vi "DriveShifter.vi"(8 "error in (no error)":errorcluster, 10 "HighGear?":bool, 11 "Pod Drive in":refnum<class "Pod Drive.lvclass">) -> (0 "error out":errorcluster, 3 "Pod Drive out":refnum<class "Pod Drive.lvclass">)   [LabVIEW 2018, in "Drive.lvlib" / "Pod Drive.lvclass"]
doc: "Shifts drive into high gear and adjusts PIDF slots"
uses:
  Pod Drive.lvclass
  Pod Drive.lvclass/Pod Drive.ctl
  Drive.lvclass
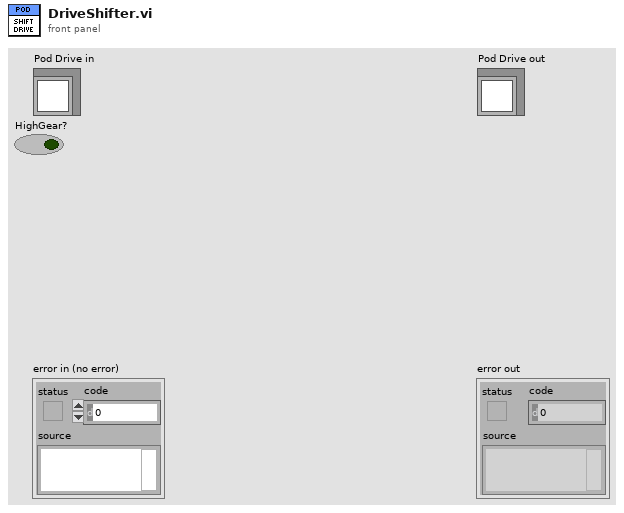
[diagram p1: front panel]
types:
  T1 = typedef "Drive.lvlib/Pod Drive.lvclass/Mode.ctl" = enum16{"ClosedLoop", "MotionMagic"}
  T2 = typedef "WPI_MotorControlDeviceRef.ctl" = cluster{"DeviceStatus":errorcluster, "Type":T3, "PWM":cluster{"PWM Channel":T4, "DeadBand":T5}, "CAN":cluster{"Device Number":u8, "SetOutput VI Ref":variant, "GetOutput VI Ref":variant, "Enable VI Ref":variant, "Disable VI Ref":variant, "Data":variant}, "Invert":bool, "DIO PWM":cluster{"PWM \"Enable\" Channel":T4, "DIOChannel":T6, "PWM Rate":dbl}}
  T3 = typedef "WPI_MotorControlType.ctl" = enum16{"PWM", "CAN", "DIO PWM"}
  T4 = typedef "FPGA_DIOPWMChannel.ctl" = enum8{"PWM 0", "PWM 1", "PWM 2", "PWM 3", "PWM 4", "PWM 5", "PWM 6", "PWM 7", "PWM 8", "PWM 9", "PWM MXP 0", "PWM MXP 1", "PWM MXP 2", "PWM MXP 3", "PWM MXP 4", "PWM MXP 5", "PWM MXP 6", "PWM MXP 7", "PWM MXP 8", "PWM MXP 9", "Invalid"}
  T5 = typedef "WPI_PWMDeadband.ctl" = cluster{"Name":string, "maxPositivePwm":i32, "minPositivePwm":i32, "centerPwm":i32, "maxNegativePwm":i32, "minNegativePwm":i32, "angularRange":u16}
  T6 = typedef "FPGA_DIOChannel.ctl" = enum8{"DIO 0", "DIO 1", "DIO 2", "DIO 3", "DIO 4", "DIO 5", "DIO 6", "DIO 7", "DIO 8", "DIO 9", "DIO MXP 0", "DIO MXP 1", "DIO MXP 2", "DIO MXP 3", "DIO MXP 4", "DIO MXP 5", "DIO MXP 6", "DIO MXP 7", "DIO MXP 8", "DIO MXP 9", "DIO MXP 10", "DIO MXP 11", "DIO MXP 12", "DIO MXP 13", "DIO MXP 14", "DIO MXP 15", "SPI Port CS1", "SPI Port CS2", "SPI Port CS3", "SPI Port MISO", "SPI Port MOSI", "Invalid"}
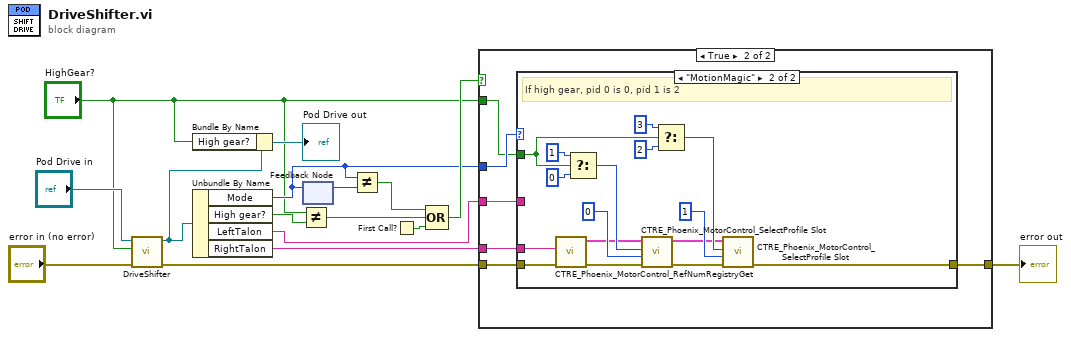
[diagram p0: block diagram]
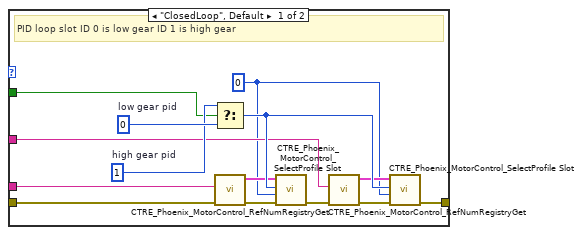
[diagram p3: hidden frame]
diagram:
  n1 = call-parent "DriveShifter.vi"("error in (no error)"="error in (no error)", "HighGear?"="HighGear?", "Drive in"="Pod Drive in") -> ("error out"=w5:errorcluster, "Drive out"=w14:refnum<class "Pod Drive.lvclass">)  [unwired: 7 in]
  n2 = Bundle By Name(cluster=w14, "High gear?"="HighGear?") -> (→"Pod Drive out":refnum<class "Pod Drive.lvclass">)
  n3 = Unbundle By Name(w14) -> ("Mode"=w9:T1, "High gear?"=w8:bool, "LeftTalon"=w6:string, "RightTalon"=w7:string)
  n4 = Not Equal?(x="HighGear?", y=w8) -> (x != y?=w11:bool)
  n5 = feedback-in #1(w9) -> ()
  n6 = feedback #1() -> (w13:T1)  [unwired: 1 in]
  n7 = Not Equal?(x=w9, y=w13) -> (x != y?=w12:bool)
  n8 = First Call?() -> (First Call?: T/F=w3:bool)
  n9 = Compound Arithmetic op=OR(w12, w11, w3) -> (w10:bool)
  n10 = case shown="True" w10 {
    tunnel: w9 -> [_ w23]
    tunnel: "HighGear?" -> [_ w22]
    tunnel: w7 -> [_ w21]
    tunnel: w6 -> [_ w20]
    tunnel: w5 -> [w17 w19]
    tunnel: [w17 w18] -> w4
    frame False {
    }
    frame True {
      n11 = case shown="\"MotionMagic\"" w23 {
        tunnel: w22 -> [w24 w51]
        tunnel: w21 -> [w29 w43]
        tunnel: w20 -> [w28 _]
        tunnel: w19 -> [w26 w39]
        tunnel: [w25 w38] -> w18
        frame "ClosedLoop", Default {
          w27 = 0 ("pidLoopIdx")
          w31 = 0  # low gear pid
          w30 = 1  # high gear pid
          # "PID loop slot ID 0 is low gear ID 1 is high gear"
          n12 = Select(t=w30, s=w24, f=w31) -> (s? t:f=w37:i32)
          n13 = call <vilib>:"CTRE_Phoenix_MotorControl_RefNumRegistryGet.vi"("error in (no error)"=w26, "refnum name"=w29) -> ("error out"=w33:errorcluster, "PhoenixMotorControlDevRef"=w34:T2)  [unwired: 8 in]
          n14 = call <vilib>:"CTRE_Phoenix_MotorControl_SelectProfile Slot.vi"("error in (no error)"=w33, "pidLoopIdx"=w27, "slotIdx"=w37, "PhoenixMotorControlDevRef"=w34) -> ("error out"=w36:errorcluster)  [unwired: 6 in, 1 out]
          n15 = call <vilib>:"CTRE_Phoenix_MotorControl_RefNumRegistryGet.vi"("error in (no error)"=w36, "refnum name"=w28) -> ("error out"=w35:errorcluster, "PhoenixMotorControlDevRef"=w32:T2)  [unwired: 8 in]
          n16 = call <vilib>:"CTRE_Phoenix_MotorControl_SelectProfile Slot.vi"("error in (no error)"=w35, "pidLoopIdx"=w27, "slotIdx"=w37, "PhoenixMotorControlDevRef"=w32) -> ("error out"=w25:errorcluster)  [unwired: 6 in, 1 out]
        }
        frame "MotionMagic" {
          # "If high gear, pid 0 is 0, pid 1 is 2"
          n17 = call <vilib>:"CTRE_Phoenix_MotorControl_RefNumRegistryGet.vi"("error in (no error)"=w39, "refnum name"=w43) -> ("error out"=w48:errorcluster, "PhoenixMotorControlDevRef"=w42:T2)  [unwired: 8 in]
          n18 = Select(t=1, s=w51, f=0) -> (s? t:f=w47:i32)
          n19 = call <vilib>:"CTRE_Phoenix_MotorControl_SelectProfile Slot.vi"("error in (no error)"=w48, "pidLoopIdx"=0, "slotIdx"=w47, "PhoenixMotorControlDevRef"=w42) -> ("error out"=w40:errorcluster, "PhoenixMotorControlDevRef"=w41:T2)  [unwired: 6 in]
          n20 = Select(t=3, s=w51, f=2) -> (s? t:f=w46:i32)
          n21 = call <vilib>:"CTRE_Phoenix_MotorControl_SelectProfile Slot.vi"("error in (no error)"=w40, "pidLoopIdx"=1, "slotIdx"=w46, "PhoenixMotorControlDevRef"=w41) -> ("error out"=w38:errorcluster)  [unwired: 6 in, 1 out]
        }
      }
    }
  }
  "error out" <- w4
